vi "Write - Download TX IQ to FPGA.vi"(0 "session in":T1[](array[typedef]) {"rx baseband session"."3630 session"."Address Space" items=["VXI/VME A16"=1, "VXI/VME A24"=2, "VXI/VME A32"=3, "VXI/VME A64"=4, "PXI Memory Allocations"=9, "PXI Configuration"=10, "PXI BAR0"=11, "PXI BAR1"=12, "PXI BAR2"=13, "PXI BAR3"=14, "PXI BAR4"=15, "PXI BAR5"=16]; "tx baseband session"."3610 session"."Address Space" items=["VXI/VME A16"=1, "VXI/VME A24"=2, "VXI/VME A32"=3, "VXI/VME A64"=4, "PXI Memory Allocations"=9, "PXI Configuration"=10, "PXI BAR0"=11, "PXI BAR1"=12, "PXI BAR2"=13, "PXI BAR3"=14, "PXI BAR4"=15, "PXI BAR5"=16]}, 5 "Wfm addr":u32, 7 "data":i16[](array[numeric]), 9 "memo":enum16{"DRAM", "BRAM"}(ring), 11 "error in":errorcluster) -> (4 "session out":T1[](array[typedef]) {"rx baseband session"."3630 session"."Address Space" items=["VXI/VME A16"=1, "VXI/VME A24"=2, "VXI/VME A32"=3, "VXI/VME A64"=4, "PXI Memory Allocations"=9, "PXI Configuration"=10, "PXI BAR0"=11, "PXI BAR1"=12, "PXI BAR2"=13, "PXI BAR3"=14, "PXI BAR4"=15, "PXI BAR5"=16]; "tx baseband session"."3610 session"."Address Space" items=["VXI/VME A16"=1, "VXI/VME A24"=2, "VXI/VME A32"=3, "VXI/VME A64"=4, "PXI Memory Allocations"=9, "PXI Configuration"=10, "PXI BAR0"=11, "PXI BAR1"=12, "PXI BAR2"=13, "PXI BAR3"=14, "PXI BAR4"=15, "PXI BAR5"=16]}, 6 "last wr addr":u32, 15 "error out":errorcluster)   [LabVIEW 2019, in "mmWave HW Control.lvlib"]
uses:
  mmWave HW Control.lvlib
  Low-level/TypeDefs/Session.ctl
  <instrlib>/niMmWave/ni3620/Config/v1/Host/Public/High-Level/niMmWave Session.ctl
  <instrlib>/_niInstr/Register Bus/v0/Host/Public/Register Bus Session.ctl
  <instrlib>/_niInstr/Register Bus/v0/Host/Private/Session Data.ctl
  <instrlib>/niMmWave/ni3620/Config/v1/Host/Public/Typedefs/Board Information.ctl
  <instrlib>/niMmWave/ni3620/Config/v1/Host/Public/Typedefs/Hardware Revision.ctl
  <instrlib>/niMmWave/ni3620/Config/v1/Host/Public/Typedefs/Gain Mapping.ctl
  <instrlib>/niMmWave/ni3620/Config/v1/Host/Public/Typedefs/Correction Data.ctl
  <instrlib>/niMmWave/ni3620/Config/v1/Host/Public/Typedefs/Opera Characterization.ctl
  <instrlib>/niMmWave/ni3620/Config/v1/Host/Public/Corrections/Typedefs/Opera Characterization Main Header.ctl
  <instrlib>/niMmWave/ni3620/Config/v1/Host/Public/Corrections/Typedefs/Opera IF Board Information.ctl
  <instrlib>/niMmWave/ni3620/Config/v1/Host/Public/Corrections/Typedefs/Opera Characterization Instance Header.ctl
  <instrlib>/niMmWave/ni3620/Config/v1/Host/Public/Corrections/Typedefs/Opera Characterization Device Data Header.ctl
  <instrlib>/niMmWave/ni3620/Config/v1/Host/Public/Corrections/Typedefs/Opera LO Characterization Data Header.ctl
  <instrlib>/niMmWave/ni3620/Config/v1/Host/Public/Corrections/Typedefs/Opera IF Board Characterization Data Header.ctl
  <instrlib>/niMmWave/ni3620/Config/v1/Host/Public/Corrections/Typedefs/Opera Characterization Device Data.ctl
  <instrlib>/niMmWave/ni3620/Config/v1/Host/Public/Corrections/Typedefs/Opera LO2 Board Characterization Data.ctl
  <instrlib>/niMmWave/ni3620/Config/v1/Host/Public/Corrections/Typedefs/Opera LO Characterization Data.ctl
  <instrlib>/niMmWave/ni3620/Config/v1/Host/Public/Corrections/Typedefs/Opera IF Board Characterization Data.ctl
  <instrlib>/niMmWave/ni3620/Config/v1/Host/Public/Corrections/Typedefs/Opera IQ Impairment Data.ctl
  <instrlib>/niMmWave/ni3620/Config/v1/Host/Public/Typedefs/mmWave Adapter Session Data.ctl
  <instrlib>/niMmWave/ni3620/Config/v1/Host/Public/Typedefs/mmWave Adapter Data.ctl
  <instrlib>/niMmWave/ni3620/Config/v1/Host/Public/Typedefs/mmWave Adapter 2.ctl
  <instrlib>/niMmWave/ni3620/Config/v1/Shared/Typedefs/Subsystem ID.ctl
  <instrlib>/niMmWave/ni3620/Config/v1/Host/Public/Typedefs/mmWave Adapter Channel Information.ctl
  <instrlib>/niMmWave/ni3620/Config/v1/Host/Public/Typedefs/Temperature Coefficients.ctl
  <instrlib>/niMmWave/ni3620/Config/v1/Host/Public/Typedefs/mmWave Characterization.ctl
  <instrlib>/niMmWave/ni3620/Config/v1/Host/Public/Corrections/Typedefs/mmWave Characterization Main Header.ctl
  <instrlib>/niMmWave/ni3620/Config/v1/Host/Public/Corrections/Typedefs/mmWave Characterization Instance Header.ctl
  <instrlib>/niMmWave/ni3620/Config/v1/Host/Public/Typedefs/Session Cache.ctl
  <instrlib>/niMmWave/ni3620/Config/v1/Host/Public/Typedefs/LO2 settings cache.ctl
  <instrlib>/niMmWave/ni3620/Config/v1/Host/Public/Typedefs/LO2 source.ctl
  <instrlib>/niMmWave/ni3620/Config/v1/Host/Public/Typedefs/Desired and Coerced.ctl
  <instrlib>/niMmWave/ni3620/Config/v1/Host/Public/Typedefs/Export cache.ctl
  <instrlib>/niMmWave/ni3620/Config/v1/Host/Public/Typedefs/Path cache.ctl
  <instrlib>/niMmWave/ni3620/Config/v1/Host/Public/Typedefs/Daughterboard Type.ctl
  <instrlib>/niMmWave/ni3620/Config/v1/Host/Public/Typedefs/LO1 settings cache.ctl
  <instrlib>/niMmWave/ni3620/Config/v1/Host/Public/Typedefs/LO1 Source.ctl
  <instrlib>/niMmWave/ni3620/Config/v1/Host/Public/Typedefs/mmWave export cache.ctl
  <instrlib>/niMmWave/ni3620/Config/v1/Host/Private/Board/LO2/LO2 Board Configuration Cache.ctl
  <instrlib>/niMmWave/ni3620/Config/v1/Host/Public/Typedefs/reference clock routing settings.ctl
  <instrlib>/niMmWave/ni3620/Config/v1/Host/Public/Typedefs/LO2 routing settings.ctl
  <instrlib>/niMmWave/ni3620/Config/v1/Host/Private/Board/LO1/LO1 Board Configuration Cache.ctl
  <instrlib>/niMmWave/ni3620/Config/v1/Host/Public/Typedefs/LO1 source settings.ctl
  <instrlib>/niMmWave/ni3620/Config/v1/Host/Public/Typedefs/LO1 export settings.ctl
  <instrlib>/niMmWave/ni3620/Config/v1/Host/Public/Typedefs/LO1 mmWave settings.ctl
  Low-level/TypeDefs/Tx Baseband Session.ctl
  <instrlib>/niMmWave/ni3610 and ni3630/controls/public/Main Settings.ctl
  <vilib>/Instr/_visa.llb/VISA Register Access Address Space.ctl
  <instrlib>/niMmWave/ni3610 and ni3630/controls/public/Register Adresses.ctl
  <instrlib>/niMmWave/ni3610 and ni3630/controls/public/Base Card Type.ctl
  <instrlib>/niMmWave/ni3610 and ni3630/controls/private/IQ Card Revision.ctl
  <instrlib>/niMmWave/ni3610 and ni3630/controls/public/Board Capability.ctl
  Low-level/TypeDefs/Blank FPGA Reference.ctl
  Low-level/TypeDefs/Rx Baseband Session.ctl
  Low-level/TypeDefs/Hardware Configuration.ctl
  Low-level/TypeDefs/Direction.ctl
  Low-level/TypeDefs/Gain Ranging.ctl
  Low-level/TypeDefs/PXI Trigger Bus Info.ctl
  Low-level/TypeDefs/TX driver FPGA ref.ctl
  <vilib>/Utility/error.llb/Error Cluster From Error Code.vi
  <vilib>/rvi/errors/niLvFpgaAdjustHostInterfaceError.vi
  <vilib>/rvi/interface/nirviMethod/nirviMethod.xnode
  <vilib>/FPGAPlugInAG/Dynamic/niLvFpga_WriteFifo_Dynamic.vi
  <vilib>/rvi/errors/niLvFpgaMergeErrorWithErrorCode.vi
  <instrlib>/_niInstr/Register Bus/v0/Host/niInstr Register Bus v0 Host.lvlib
  <instrlib>/niMmWave/ni3610 and ni3630/ni3610_and_ni3630_Driver_Lib.lvlib
  <instrlib>/niMmWave/ni3620/Config/v1/Host/niMmWave Config v1 Host.lvlib
  <instrlib>/niMmWave/ni3620/Config/v1/Shared/niMmWave Config v1 Shared.lvlib
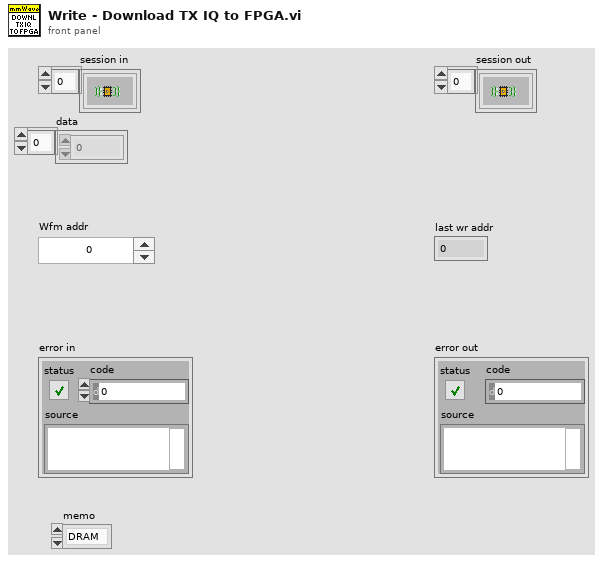
[diagram p1: front panel]
types:
  T1 = typedef "Session.ctl" = cluster{"3620 session":refnum<queue>, "tx baseband session":T2, "rx baseband session":T10, "tx gain (dB)":dbl, "rx gain (dB)":dbl, "hardware configuration":T11, "gain ranging":T13[], "pxi trigger bus information":T14}
  T2 = typedef "Tx Baseband Session.ctl" = cluster{"3610 session":T3, "7902 reference":T9}
  T3 = typedef "ni3610_and_ni3630_Driver_Lib.lvlib/Main Settings.ctl" = cluster{"VISA resource name":refnum<visa-resource-name>, "Address Space":T4, "window_offset":u32, "register_addresses":T5, "required_MM_fpga_version":cluster{"signature":u32, "hardware":u32, "current revision":u32, "oldest revision":u32}, "CPLD Oldest Compat Version ":cluster{"hardware":u32, "CPLD firmware":u32}, "MM_FPGA_image_location":string, "is_init":bool, "card_type":T6, "DacLmkConfigFileName":string, "AdcLmkConfigFileName":string, "AdcConfigFileName":string, "DacConfigFileName_RevA":string, "DacConfigFileName_RevB":string, "Mulde hardware revision":u8, "bypass DAC PLL\n":bool, "IQ Card Revision":T7, "board capability":T8}
  T4 = typedef "VISA Register Access Address Space.ctl" = u16
  T5 = typedef "ni3610_and_ni3630_Driver_Lib.lvlib/Register Adresses.ctl" = cluster{"MM based Registers":cluster{"Revision":u32, "OldestCompatRev":u32, "signature":u32, "scratch":u32, "LedControl":u32, "BoardHwRev":u32, "BoardControl":u32, "ThermalStatus":u32, "BasebandStatus":u32, "BasebandControl":u32, "BasebandAuxSetup":u32, "BasebandAuxStatus":u32, "LmkSyncOutSetup":u32, " AdcSyncOutSetup":u32, " InjSyncOutSetup":u32, " PxiTrig0OutSetup":u32, " PxiTrig1OutSetup":u32, " PxiTrig2OutSetup":u32, " PxiTrig3OutSetup":u32, " PxiTrig4OutSetup":u32, " PxiTrig5OutSetup":u32, " PxiTrig6OutSetup":u32, " PxiTrig7OutSetup":u32}, "CPLD based Registers":cluster{"SlaveSignature":u32, "SlaveRevision":u32, "SlaveOldestCompatRev":u32, "SlaveScratch":u32, "SlaveSetup":u32, "SlaveStatus":u32, "IDacReg_offset":u32, "LMKRegGrp0_offset":u32, "QDacReg_offset":u32, "BrdTempSensorVal":u32, "TempSensorPowerDown":u32, "GPIOReg_offset":u32, "IAdcReg_offset":u32, "QAdcReg_offset":u32, "LMKRegGrp1_offset":u32, "QadcTempSensorVal":u32, "IadcTempSensorVal":u32, "RevisionReg":u32, "VcxoReg":u32, "CpldStatusReg":u32, "PowerReg":u32, "VBiasEnReg":u32, "ExtRefOeReg":u32, "QdacCtrlReg":u32, "QdacStatusReg":u32, "IdacCtrlReg":u32, "IdacStatusReg":u32, "QdacJtagIn":u32, "QdacJtagOut":u32, "IdacJtagIn":u32, "IdacJtagOut":u32, "IqDcSetupReg":u32, "QadcStatusReg":u32, "IadcStatusReg":u32, "BrdSetupReg":u32, "IqDcRevisionReg":u32, "PllStatusReg":u32, "EndpointScratchReg":u32, "AdcSyncCfgReg":u32, "IqCardOpampReg":u32}, "CPLD Register Offset":u32, "MM  Register Offset":u32, " PxiTrig0OutSetup":u32}
  T6 = typedef "ni3610_and_ni3630_Driver_Lib.lvlib/Base Card Type.ctl" = enum16{"unspecified", "ADC", "DAC"}
  T7 = typedef "ni3610_and_ni3630_Driver_Lib.lvlib/IQ Card Revision.ctl" = enum16{"RevA", "RevB", "RevC", "RevD"}
  T8 = typedef "ni3610_and_ni3630_Driver_Lib.lvlib/Board Capability.ctl" = cluster{"baseband sync":enum16{"no baseband sync", "baseband sync"}}
  T9 = typedef "Blank FPGA Reference.ctl" = refnum<k20>
  T10 = typedef "Rx Baseband Session.ctl" = cluster{"3630 session":T3, "7902 reference":T9}
  T11 = typedef "Hardware Configuration.ctl" = cluster{"direction":T12, "baseband only":bool}
  T12 = typedef "Direction.ctl" = enum16{"Transceiver", "Receiver", "Transmitter"}
  T13 = typedef "Gain Ranging.ctl" = cluster{"gain ranging active scope":string, "gain ranging stream session":refnum<k20>}
  T14 = typedef "PXI Trigger Bus Info.ctl" = cluster{"chassis resource name":refnum<visa-resource-name>, "7902R (TX)":i16, "3610 (TX)":i16, "3620 (IF)":i16, "3630 (RX)":i16, "7902R (RX)":i16}
  T15 = typedef "TX driver FPGA ref.ctl" = refnum<k20>
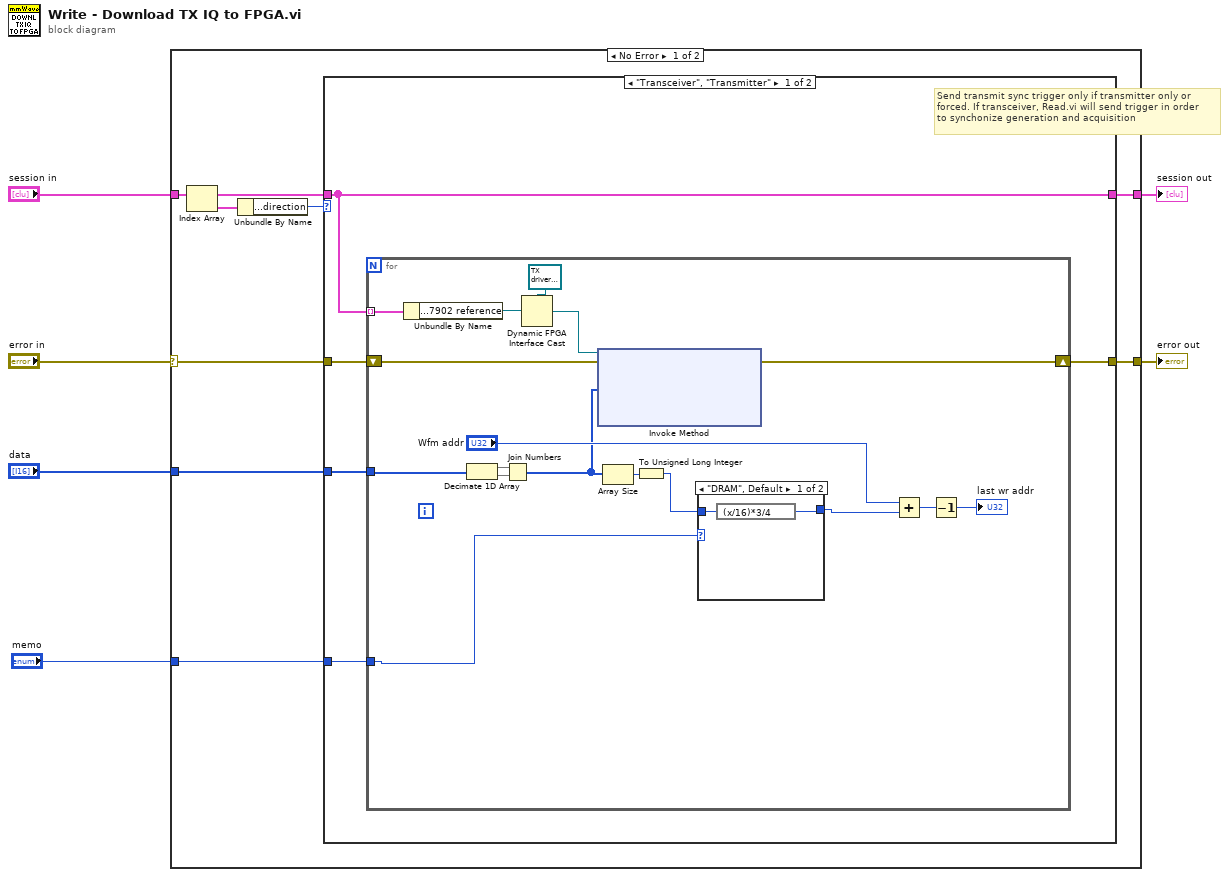
[diagram p0: block diagram]
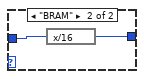
[diagram p2: hidden frame]
diagram:
  n1 = case shown="No Error" "error in" {
    selector: "error in" -> [w14 w44]
    tunnel: "session in" -> [w12 w43]
    tunnel: [w13 w44] -> w5
    tunnel: [w9 w43] -> w3
    tunnel: "data" -> [w8 _]
    tunnel: "memo" -> [w7 _]
    frame No Error {
      n2 = Index Array(array=w12) -> (element=w11:T1)  [unwired: 1 in]
      n3 = Unbundle By Name(w11) -> ("hardware configuration.direction"=w10:T12)
      n4 = case shown="\"Transceiver\", \"Transmitter\"" w10 {
        tunnel: w14 -> [w19 w42]
        tunnel: [w18 w42] -> w13
        tunnel: w12 -> [w17 w41]
        tunnel: [w17 w41] -> w9
        tunnel: w8 -> [w16 _]
        tunnel: w7 -> [w15 _]
        frame "Transceiver", "Transmitter" {
          # "Send transmit sync trigger only if transmitter only or\nforced. If transceiver, Read.vi will send trigger in order\nto synchonize generation and acquisition"
          n5 = for {
            shift-right: [w31] -> w18
            shift-left: w19 -> [w22]
            tunnel: w17 -> [w36] mode=indexing
            tunnel: w16 -> [w20]
            tunnel: w15 -> [w27]
            n6 = Unbundle By Name(w36) -> ("tx baseband session.7902 reference"=w35:T9)
            n7 = Decimate 1D Array(w20) -> (w25:i16[], w24:i16[])
            n8 = Join Numbers(hi=w25, lo=w24) -> ((hi.lo)=w26:u32[])
            n9 = Dynamic FPGA Interface Cast(Session In=T15 refnum ("TX FPGA ref"), Type=w35) -> (Session Out=w23:T15)
            n10 = xnode "Invoke Method"("FPGA VI Reference In"=w23, "error in"=w22, "Data"=w26) -> ("error out"=w31:errorcluster)  [unwired: 1 in, 2 out]
            n11 = Array Size(array=w26) -> (size(s)=w33:i32)
            n12 = To Unsigned Long Integer(number=w33) -> (unsigned 32bit integer=w29:u32)
            n13 = case shown="\"DRAM\", Default" w27 {
              tunnel: w29 -> [w38 w40]
              tunnel: [w37 w39] -> w28
              frame "DRAM", Default {
                n14 = expression code="(x/16)*3/4"(w38) -> (w37:u32)
              }
              frame "BRAM" {
                n15 = expression code="x/16"(w40) -> (w39:u32)
              }
            }
            n16 = Add(x="Wfm addr", y=w28) -> (x+y=w30:u32)
            n17 = Decrement(x=w30) -> (x-1=→"last wr addr":u32)
          }
        }
        frame "Receiver" {
        }
      }
    }
    frame Error {
    }
  }
  "session out" <- w3
  "error out" <- w5
